vi "Write File.vi"(8 "error in (no error)":errorcluster, 11 "[Data] Userinfo Binary in":refnum<class "[Data] Userinfo Binary.lvclass">) -> (0 "error out":errorcluster, 3 "[Data] Userinfo Binary out":refnum<class "[Data] Userinfo Binary.lvclass">)   [LabVIEW 2020, in "[Data] Userinfo Binary.lvclass"]
uses:
  [Data] Userinfo Binary.lvclass
  [Data] Userinfo Binary.lvclass/[Data] Userinfo Binary.ctl
  <vilib>/YU/YU-Encrypt/AES/AES.lvclass
  <vilib>/YU/YU-Encrypt/Base64/Base64.lvclass
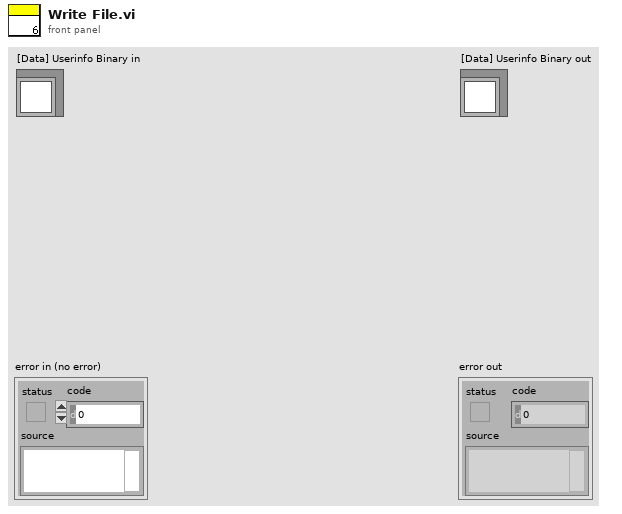
[diagram p1: front panel]
types:
  T1 = enum16{"open", "replace", "create", "open or create", "replace or create", "replace or create with confirmation"}
  T2 = typedef "[Data] Userinfo Binary.lvclass/user info.ctl" = cluster{"password":string, "authority":i8, "department":string, "post":string, "remark":string, "create time":string, "last login time":string}
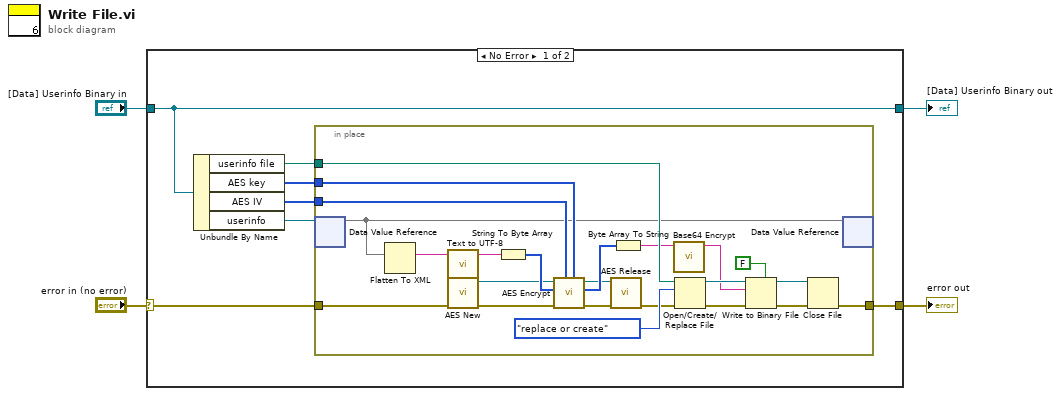
[diagram p0: block diagram]
diagram:
  n1 = case shown="No Error" "error in (no error)" {
    selector: "error in (no error)" -> [w5 w36]
    tunnel: [w7 w36] -> w3
    tunnel: [w11 w35] -> w1
    tunnel: "[Data] Userinfo Binary in" -> [w11 w35]
    frame No Error {
      n2 = Unbundle By Name(w11) -> ("userinfo file"=w8:path, "AES key"=w10:u8[], "AES IV"=w9:u8[], "userinfo"=w6:refnum<data-value>)
      n3 = in-place {
        in-place-border: w10 -> [w30]
        in-place-border: w9 -> [w29]
        in-place-border: w8 -> [w27]
        in-place-border: [w21] -> w7
        in-place-border: w5 -> [w14]
        n4 = in-place-dvr #1(w6) -> (w12:map{string, T2})  [unwired: 1 out]
        n5 = Flatten To XML(6:w12) -> (2:w13:string)
        n6 = call <vilib>:"Text to UTF-8.vi"("text"=w13) -> ("utf-8 text"=w33:string)  [unwired: 4 in]
        n7 = call <vilib>:"AES New.vi"("error in (no error)"=w14) -> ("error out"=w34:errorcluster, "AES out"=w31:refnum<class "AES.lvclass">)  [unwired: 9 in]
        n8 = String To Byte Array(string=w33) -> (unsigned byte array=w32:u8[])
        n9 = call <vilib>:"AES Encrypt.vi"("Key"=w30, "IV"=w29, "error in (no error)"=w34, "data"=w32, "AES in"=w31) -> ("error out"=w20:errorcluster, "encrypted data"=w28:u8[], "AES out"=w19:refnum<class "AES.lvclass">)  [unwired: 4 in]
        n10 = call <vilib>:"AES Release.vi"("error in (no error)"=w20, "AES in"=w19) -> ("error out"=w18:errorcluster)  [unwired: 9 in]
        n11 = Byte Array To String(unsigned byte array=w28) -> (string=w16:string)
        n12 = call <vilib>:"Base64 Encrypt.vi"("data"=w16) -> ("encrypted data"=w15:string)  [unwired: 9 in, 1 out]
        n13 = Open/Create/Replace File(file path (use dialog)=w27, error in=w18, operation (0:open)=T1."replace or create") -> (refnum out=w24:refnum<file>, error out=w25:errorcluster)  [unwired: 3 in, 1 out]
        n14 = Write to Binary File(file (use dialog)=w24, data=w15, error in=w25, 5:FALSE ("prepend array or string size? (T)")) -> (refnum out=w22:refnum<file>, error out=w23:errorcluster)  [unwired: 2 in, 1 out]
        n15 = Close File(refnum=w22, error in=w23) -> (error out=w21:errorcluster)  [unwired: 1 out]
        n16 = in-place-dvr #1(w12) -> ()  [unwired: 2 out]
      }
    }
    frame Error {
    }
  }
  "error out" <- w3
  "[Data] Userinfo Binary out" <- w1
